vi "CleanupString.vi"(11 "Input String":string) -> (3 "Output String":string)   [LabVIEW 2019, in "LabErrorUX.lvclass"]
doc: "Trim whitespace and replace end of line with line feed constant to standardize"
uses:
  LabErrorUX.lvclass
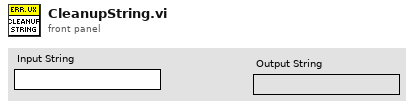
[diagram p1: front panel]
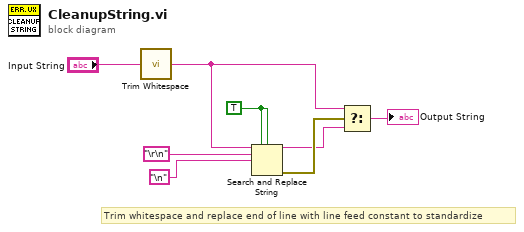
[diagram p0: block diagram]
diagram:
  w7 = TRUE ("replace all? (F)")
  # "Trim whitespace and replace end of line with line feed constant to standardize"
  n1 = call <vilib>:"Trim Whitespace.vi"("string"="Input String") -> ("trimmed string"=w3:string)  [unwired: 1 in]
  n2 = Search and Replace String(replace all?=w7, case sensitive?=w7, input string=w3, search string="\r\n", replace string="\n") -> (result string=w2:string, error out=w4:errorcluster)  [unwired: 3 in, 2 out]
  n3 = Select(t=w3, s=w4, f=w2) -> (s? t:f=→"Output String":string)
